vi "OfflineTrackerHandleMVL2.vi"(4 "error in":errorcluster, 5 "action":enum16{"get", "set"}(ring), 6 "in":T2={"front panel settings"={"files"={"LUT path"=path "", "Trace path"=path "", " folders #"=0, "base path"=path "", "use trace"=FALSE, "use base"=FALSE, "LUT tmp"=0, "Trace tmp"=0, "active path"=path ""}, "Tracking"={"RminZ (pix)"=0, "Rmax (pix)"=0, "angular pixel \ncoverage factor"=0.0, "radial pixel \ncoverage factor"=0.0}, "Frames"={"Start frame"=0, "number of frames"=0, "display frame "=0, "track every nd frame "=0, "Track all frames"=FALSE, "active frame"=0}, "Calibs"={"Zlut number of steps"=0, "pix/um"=0.0, "Z correction factor"=0.0, "Zlut step size (um)"=0.0, "ROI(pix)"=0}, "Beads"={"number of ref beads"=0, "overlay"=FALSE}, "Misc"={"save images to new location"=FALSE, "destination"=path ""}}, "data"={"Image"="Image", "image size"=[], "Bead Array"=[], "overlay image"=refnum, "# beads"=0, "Job list"=[], "job running"=FALSE, "job #"=0, "folders to go"=0}}) -> (0 "error out":errorcluster, 2 "out":T2={"front panel settings"={"files"={"LUT path"=path "", "Trace path"=path "", " folders #"=0, "base path"=path "", "use trace"=FALSE, "use base"=FALSE, "LUT tmp"=0, "Trace tmp"=0, "active path"=path ""}, "Tracking"={"RminZ (pix)"=0, "Rmax (pix)"=0, "angular pixel \ncoverage factor"=0.0, "radial pixel \ncoverage factor"=0.0}, "Frames"={"Start frame"=0, "number of frames"=0, "display frame "=0, "track every nd frame "=0, "Track all frames"=FALSE, "active frame"=0}, "Calibs"={"Zlut number of steps"=0, "pix/um"=0.0, "Z correction factor"=0.0, "Zlut step size (um)"=0.0, "ROI(pix)"=0}, "Beads"={"number of ref beads"=0, "overlay"=FALSE}, "Misc"={"save images to new location"=FALSE, "destination"=path ""}}, "data"={"Image"="Image", "image size"=[], "Bead Array"=[], "overlay image"=refnum, "# beads"=0, "Job list"=[], "job running"=FALSE, "job #"=0, "folders to go"=0}})   [LabVIEW 2011]
uses:
  <vilib>/vision/Image Controls.llb/IMAQ Image.ctl
panel:
  in  "FirstimageName":path=path "D:/mtjvanloenhout/Desktop/tracking/40x/tmp_133"
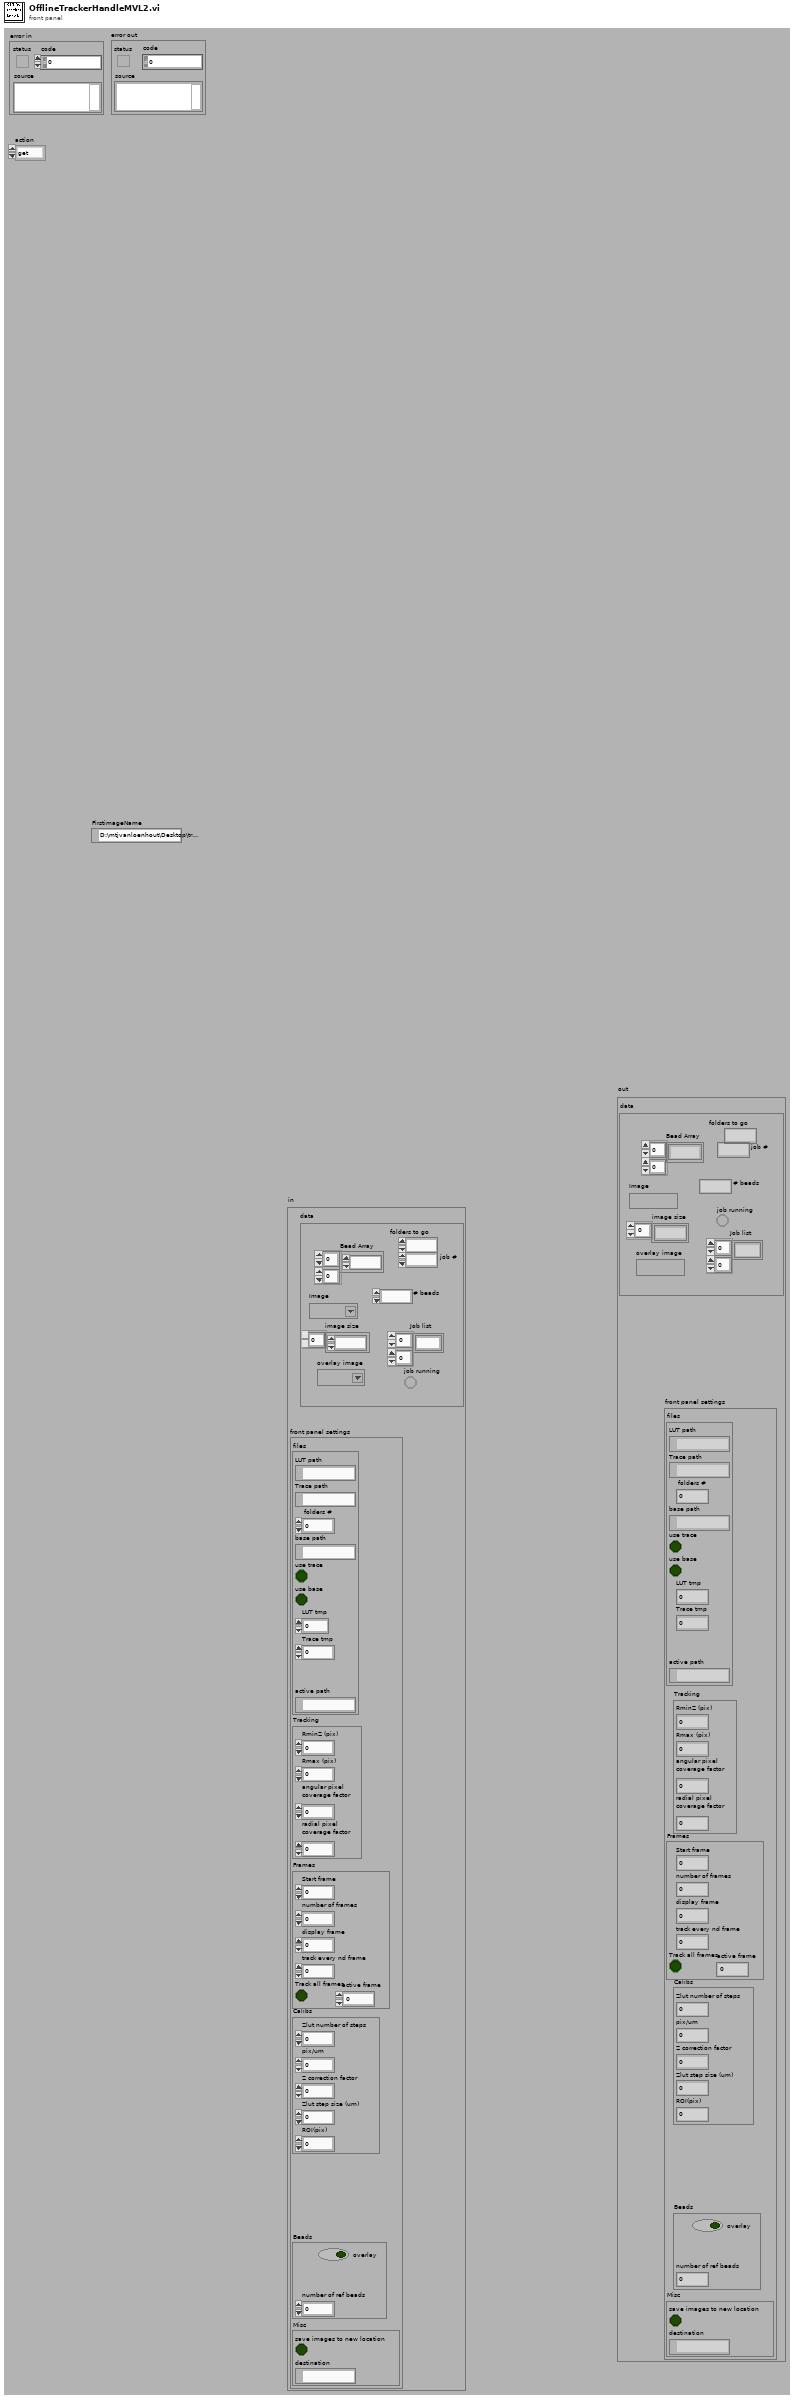
[diagram p1: front panel]
types:
  T1 = typedef "IMAQ Image.ctl" = refnum<image>
  T2 = cluster{"front panel settings":cluster{"files":cluster{"LUT path":path, "Trace path":path, " folders #":i32, "base path":path, "use trace":bool, "use base":bool, "LUT tmp":i32, "Trace tmp":i32, "active path":path}, "Tracking":cluster{"RminZ (pix)":i32, "Rmax (pix)":i32, "angular pixel \ncoverage factor":dbl, "radial pixel \ncoverage factor":dbl}, "Frames":cluster{"Start frame":i32, "number of frames":u32, "display frame ":i32, "track every nd frame ":i32, "Track all frames":bool, "active frame":i32}, "Calibs":cluster{"Zlut number of steps":i32, "pix/um":dbl, "Z correction factor":dbl, "Zlut step size (um)":dbl, "ROI(pix)":i32}, "Beads":cluster{"number of ref beads":i32, "overlay":bool}, "Misc":cluster{"save images to new location":bool, "destination":path}}, "data":cluster{"Image":T1, "image size":i32[], "Bead Array":i32[][], "overlay image":T1, "# beads":i32, "Job list":string[][], "job running":bool, "job #":i32, "folders to go":i32}}
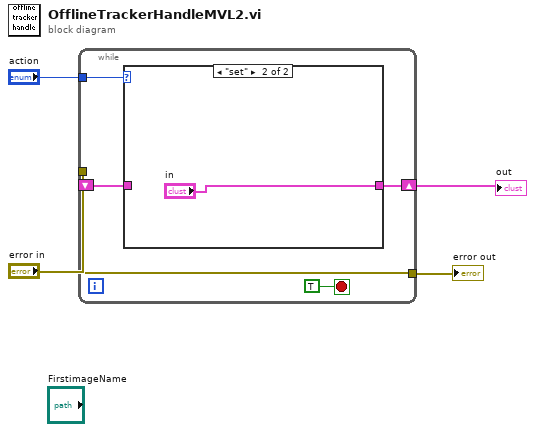
[diagram p0: block diagram]
diagram:
  n1 = while {
    tunnel: "error in" -> [w8]
    tunnel: [w8] -> w2
    tunnel: "action" -> [w7]
    shift-right: [w6] -> w1
    shift-left: _ -> [w5]
    stop <- TRUE ("stop") stop-if-true
    n2 = case shown="\"set\"" w7 {
      tunnel: [w10 "in"] -> w6
      tunnel: w5 -> [w10 _]
      frame "get" {
      }
      frame "set" {
      }
    }
  }
  "error out" <- w2
  "out" <- w1
